vi "GlobalVariables.vi"() -> ()   [LabVIEW 2009, in "Keithley 2600 Series.lvlib"]
uses:
  <instrlib>/Keithley 2600 Series/Keithley 2600 Series.lvlib
panel:
  in  "Error Query":bool=TRUE
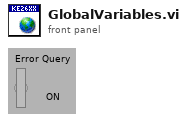
[diagram p1: front panel]
diagram:
